vi "LSMcontroller_v62_updatedpointscan.vi"() -> ()   [LabVIEW 2015] (continued)
                                n1697 = call "calib.vi"() -> ()  [unwired: 1 in]
                                }
                                frame #2 {
                                n1698 = call "setup.vi"() -> ()  [unwired: 1 in]
                                }
                                }
                                }
                                }
                              }
                              frame Enabled {
                              }
                            }
                            n1699 = local write "64bit disabled"(TRUE ("64bit disabled")) -> ()
                          }
                          frame #2 {
                            n1700 = local read "save\ndata"() -> (w4480:bool)
                            n1701 = case shown="True" w4480 {
                              tunnel: w4481 -> [_ w4485]
                              frame False {
                              }
                              frame True {
                                n1702 = local read "filename prefix"() -> (w4483:string)
                                n1703 = local read "data dir"() -> (w4484:path)
                                n1704 = call "preparebinaryfiles.vi"("filename prefix"=w4483, "data dir"=w4484, "timestamp"=w4485) -> ("full-filename"=w4482:string)  [unwired: 1 in]
                                n1705 = local write "full-filename"(w4482) -> ()
                              }
                            }
                            n1706 = call "preptempbuffers_tt.vi"() -> ()  [unwired: 12 in]
                          }
                          frame #3 {
                            n1707 = local read "wavdet"() -> (w4486:bool)
                            n1708 = case shown="False" w4486 {
                              frame False {
                                n1709 = disable-structure shown="Disabled" {
                                frame Disabled {
                                n1710 = call "2pparameters.vi"("command"="get") -> ("params out"=w4488:T10)  [unwired: 1 in]
                                n1711 = Unbundle By Name(w4488) -> ("autoshutter"=w4489:bool)
                                n1712 = case shown="True" w4489 {
                                frame False {
                                }
                                frame True {
                                n1713 = call "shuttercontrol.vi"("command"="open") -> ()  [unwired: 1 in, 1 out]
                                }
                                }
                                }
                                frame Enabled {
                                }
                                }
                              }
                              frame True {
                              }
                            }
                          }
                          frame #4 {
                            n1714 = flat-sequence {
                              frame #0 {
                                # "Disabled for conversion to 64 bit"
                                n1715 = disable-structure shown="Disabled" {
                                frame Disabled {
                                n1716 = local read "Measurement"() -> (w4492:T4)
                                n1717 = case shown="\"Lifetime (contour)\"" w4492 {
                                frame "X-Y-t movie", Default {
                                }
                                frame "Lifetime (contour)" {
                                n1718 = call "runLT_img.vi"() -> ()  [unwired: 1 in]
                                }
                                }
                                }
                                frame Enabled {
                                }
                                }
                                n1719 = local write "64bit disabled"(TRUE ("64bit disabled")) -> ()
                              }
                              frame #1 {
                                n1720 = call "runAI_img.vi"() -> ()  [unwired: 12 in]
                                n1721 = call "runCI.vi"() -> ()  [unwired: 12 in]
                                n1722 = call "runDO_img.vi"() -> ()  [unwired: 12 in]
                              }
                              frame #2 {
                                n1723 = call "runAO_img.vi"() -> ()  [unwired: 12 in]
                              }
                            }
                          }
                          frame #5 {
                            # "Disabled for conversion to 64 bit"
                            n1724 = disable-structure shown="Disabled" {
                              disable-tunnel: w4494 -> [w4495 _]
                              frame Disabled {
                                w4498 = u16 0 items=["Stream to disk", "Post process", "real time process"] ("Ring")
                                n1725 = local read "T3R Data processing"() -> (w4497:u16)
                                n1726 = Equal?(x=w4497, y=w4498) -> (x = y?=w4496:bool)
                                n1727 = local read "save\ndata"() -> (w4500:bool)
                                n1728 = local read "Measurement"() -> (w4501:T4)
                                n1729 = And(x=w4500, y=w4496) -> (x .and. y?=w4499:bool)
                                n1730 = case shown="\"Lifetime (contour)\"" w4501 {
                                tunnel: w4495 -> [_ w4505]
                                tunnel: w4499 -> [_ w4503]
                                frame "X-Y-t movie", Default {
                                }
                                frame "Lifetime (contour)" {
                                n1731 = case shown="True" w4503 {
                                selector: w4503 -> [w4506 w4511]
                                tunnel: w4505 -> [_ w4509]
                                tunnel: [path "" ("appended path") w4512] -> w4504
                                tunnel: [w4506 w4511] -> w4502
                                frame False {
                                }
                                frame True {
                                n1732 = local read "filename prefix"() -> (w4510:string)
                                n1733 = local read "data dir"() -> (w4513:path)
                                n1734 = call "generatedatafilename.vi"("timestamp"=w4509, "filename prefix in"=w4510) -> ("full-filename"=w4508:string)
                                n1735 = Concatenate Strings(w4508, ".lvpt3contour" ("string")) -> (w4515:string)
                                n1736 = Build Path(base path=w4513, name or relative path=w4515) -> (appended path=w4512:path)
                                }
                                }
                                n1737 = call "collectLT_res_v1.vi"("stream?"=w4502, "data file"=w4504) -> ()  [unwired: 2 out]
                                }
                                }
                              }
                              frame Enabled {
                              }
                            }
                            n1738 = while {
                              i -> [w4518]
                              stop <- w4516 stop-if-true
                              n1739 = local read "Stop"() -> (w4526:bool)
                              n1740 = local read "Exit"() -> (w4525:bool)
                              n1741 = Increment(x=w4518) -> (x+1=w4517:i32)
                              n1742 = local write "points recorded"(w4517) -> ()
                              n1743 = Or(x=w4526, y=w4525) -> (x .or. y?=w4524:bool)
                              n1744 = case shown="False" w4524 {
                                frame False {
                                n1745 = stacked-sequence {
                                frame #0 {
                                n1746 = call "collectAI_tt_V2.vi"() -> ()  [unwired: 4 in]
                                n1747 = call "collectCI_tt.vi"() -> ("size(s)"=w4533:i32)  [unwired: 3 in]
                                n1748 = local write "scol"(w4533) -> ()
                                }
                                frame #1 {
                                n1749 = local read "Live"() -> (w4534:bool)
                                n1750 = case shown="True" w4534 {
                                frame False {
                                }
                                frame True {
                                n1751 = local read "graph1list"() -> (w4541:u16)
                                n1752 = local read "graph2list"() -> (w4540:u16)
                                n1753 = To Unsigned Word Integer(number=w4541) -> (unsigned 16bit integer=w4539:u16)
                                n1754 = To Unsigned Word Integer(number=w4540) -> (unsigned 16bit integer=w4538:u16)
                                n1755 = call "dattotrace.vi"("graph2list"=w4538, "Current Average"=sgl 1.0, "graph1list"=w4539) -> ("trace2array out"=w4536:sgl[], "trace1array out"=w4547:sgl[])
                                n1756 = local read "bin"() -> (w4548:dbl)
                                n1757 = script code="data=reshape(datain,[bin length(datain)./bin]);\ndataout=mean(data,1);\ndata2=reshape(datain2,[bin length(datain2)./bin]);\ndataout2=mean(data2,1);"("bin"=w4548, "datain"=w4547, "datain2"=w4536) -> ("dataout"=w4546:dbl[], "dataout2"=w4535:dbl[])  [unwired: 1 in, 1 out]
                                n1758 = Array Size(array=w4535) -> (size(s)=w4549:i32)
                                n1759 = Divide(x=w4549, y=2) -> (x/y=w4551:dbl)
                                n1760 = Round To Nearest(number=w4551) -> (nearest integer value=w4553:dbl)
                                n1761 = Array Size(array=w4546) -> (size(s)=w4558:i32)
                                n1762 = Delete From Array(array=w4535, length=w4553, index=0) -> (deleted portion=w4544:dbl[], array with subset deleted=w4545:dbl[])
                                n1763 = Divide(x=w4558, y=2) -> (x/y=w4556:dbl)
                                n1764 = Round To Nearest(number=w4556) -> (nearest integer value=w4554:dbl)
                                n1765 = Delete From Array(array=w4546, length=w4554, index=0) -> (deleted portion=w4543:dbl[], array with subset deleted=w4542:dbl[])
                                n1766 = local write "graph2"(w4542) -> ()
                                n1767 = local write "graph1"(w4543) -> ()
                                n1768 = local write "graph3"(w4544) -> ()
                                n1769 = local write "graph4"(w4545) -> ()
                                }
                                }
                                }
                                frame #2 {
                                n1770 = local read "save\ndata"() -> (w4559:bool)
                                n1771 = case shown="True" w4559 {
                                frame False {
                                }
                                frame True {
                                n1772 = call "savebinaryfiles.vi"() -> ()  [unwired: 1 in]
                                }
                                }
                                }
                                }
                                }
                                frame True {
                                }
                              }
                              n1773 = local read "continuous"() -> (w4521:bool)
                              n1774 = case shown="False" w4521 {
                                tunnel: w4517 -> [w4531 _]
                                tunnel: [w4530 FALSE] -> w4519
                                frame False {
                                n1775 = call "2pparameters.vi"("command"="get") -> ("params out"=w4528:T10)  [unwired: 1 in]
                                n1776 = Unbundle By Name(w4528) -> ("tt_cycles"=w4527:i32)
                                n1777 = Greater Or Equal?(x=w4531, y=w4527) -> (x >= y?=w4530:bool)
                                }
                                frame True {
                                }
                              }
                              n1778 = local read "Stop"() -> (w4523:bool)
                              n1779 = local read "Exit"() -> (w4522:bool)
                              n1780 = Or(x=w4523, y=w4522) -> (x .or. y?=w4520:bool)
                              n1781 = Or(x=w4520, y=w4519) -> (x .or. y?=w4516:bool)
                            }
                            n1782 = local write "64bit disabled"(TRUE ("64bit disabled")) -> ()
                          }
                          frame #6 {
                            # "Disabled for conversion to 64 bit"
                            n1783 = local read "Measurement"() -> (w4562:T4)
                            n1784 = disable-structure shown="Disabled" {
                              disable-tunnel: w4562 -> [w4564 _]
                              disable-tunnel: w4561 -> [w4563 _]
                              frame Disabled {
                                n1785 = case shown="\"Lifetime (contour)\"" w4564 {
                                tunnel: w4563 -> [_ w4565]
                                frame "X-Y-t movie", Default {
                                }
                                frame "Lifetime (contour)" {
                                n1786 = stacked-sequence {
                                tunnel: w4565 -> [_ w4566]
                                frame #0 {
                                n1787 = flat-sequence {
                                frame #0 {
                                n1788 = call "stoperaseLT_img.vi"() -> ()  [unwired: 1 in]
                                }
                                }
                                }
                                frame #1 {
                                w4569 = u16 0 items=["Stream to disk", "Post process", "real time process"] ("Ring")
                                n1789 = local read "T3R Data processing"() -> (w4568:u16)
                                n1790 = local read "save\ndata"() -> (w4571:bool)
                                n1791 = Equal?(x=w4568, y=w4569) -> (x = y?=w4567:bool)
                                n1792 = Not(x=w4567) -> (.not. x?=w4572:bool)
                                n1793 = And(x=w4571, y=w4572) -> (x .and. y?=w4570:bool)
                                n1794 = case shown="True" w4570 {
                                tunnel: w4566 -> [_ w4573]
                                frame False {
                                }
                                frame True {
                                n1795 = local read "filename prefix"() -> (w4574:string)
                                n1796 = local read "data dir"() -> (w4590:path)
                                n1797 = call "2pparameters.vi"("command"="get") -> ("params out"=w4585:T10)  [unwired: 1 in]
                                n1798 = call "generatedatafilename.vi"("timestamp"=w4573, "filename prefix in"=w4574) -> ("full-filename"=w4575:string)
                                n1799 = Unbundle By Name(w4585) -> ("srate"=w4583:sgl, "Pel"=w4582:sgl, "measpoints"=w4580:i32)
                                n1800 = Concatenate Strings(w4575, ".lvpt3contour" ("string")) -> (w4588:string)
                                n1801 = Build Path(base path=w4590, name or relative path=w4588) -> (appended path=w4587:path)
                                n1802 = To Unsigned Long Integer(number=w4583) -> (unsigned 32bit integer=w4584:u32)
                                n1803 = To Unsigned Long Integer(number=w4582) -> (unsigned 32bit integer=w4581:u32)
                                n1804 = To Unsigned Long Integer(number=w4580) -> (unsigned 32bit integer=w4579:u32)
                                n1805 = call "PH-temp-raw.vi"("command"="get") -> ("array out"=w4578:u32[])  [unwired: 1 in]
                                n1806 = Build Array (concatenate)(w4584, w4581, w4579, w4578) -> (w4577:u32[])
                                n1807 = Open/Create/Replace File(file path (use dialog)=w4587, operation (0:open)=T8."replace or create") -> (refnum out=w4594:refnum<file>, error out=w4593:errorcluster)  [unwired: 4 in, 1 out]
                                n1808 = Write to Binary File(file (use dialog)=w4594, data=w4577, error in=w4593, 5:FALSE ("prepend array or string size? (T)")) -> (refnum out=w4591:refnum<file>, error out=w4592:errorcluster)  [unwired: 2 in, 1 out]
                                n1809 = Close File(refnum=w4591, error in=w4592) -> ()  [unwired: 2 out]
                                }
                                }
                                }
                                }
                                }
                                }
                              }
                              frame Enabled {
                              }
                            }
                            n1810 = local write "64bit disabled"(TRUE ("64bit disabled")) -> ()
                          }
                          frame #7 {
                            n1811 = call "reset AO_DO_v3.vi"() -> ()  [unwired: 12 in]
                          }
                          frame #8 {
                            n1812 = stacked-sequence {
                              tunnel: w4610 -> [w4613 _ _ _ _ _]
                              tunnel: w4607 -> [w4612 _ _ _ _ _]
                              tunnel: w4608 -> [w4611 _ _ _ _ _]
                              tunnel: w4609 -> [_ w4662 _ _ _ _]
                              tunnel: w4605 -> [_ w4661 w4716 w4813 _ _]
                              tunnel: w4606 -> [_ w4660 w4715 w4812 _ _]
                              tunnel: w4604 -> [_ _ _ w4811 _ _]
                              tunnel: w4603 -> [_ _ _ w4810 _ _]
                              tunnel: w4602 -> [_ _ w4713 _ _ _]
                              tunnel: w4601 -> [_ _ w4712 _ _ _]
                              tunnel: w4600 -> [_ _ w4710 _ _ _]
                              tunnel: w4599 -> [_ _ w4709 _ _ _]
                              tunnel: w4598 -> [_ _ _ w4808 _ _]
                              tunnel: w4597 -> [_ _ _ w4807 _ _]
                              frame #0 {
                                n1813 = case shown="False" w4613 {
                                tunnel: w4612 -> [_ w4635]
                                tunnel: w4611 -> [_ w4634]
                                frame True {
                                n1814 = stacked-sequence {
                                seq-local: [w4614 _ _] -> [_ w4626 w4631]
                                frame #0 {
                                n1815 = call "configuration.vi"("command"="get") -> ("config out"=w4620:T11)  [unwired: 2 in, 1 out]
                                n1816 = Unbundle By Name(w4620) -> ("Voltage to Xgalvo"=w4617:i32)
                                n1817 = call "2pparameters.vi"("command"="get") -> ("params out"=w4618:T10)  [unwired: 1 in]
                                n1818 = in-place {
                                in-place-border: w4617 -> [w4625]
                                in-place-border: [w4622] -> w4614
                                n1819 = in-place-cluster #31(w4618) -> ("aAO"=w4624:u32[])
                                n1820 = call "remove channel from active arrayv2.vi"("line array in"=w4624, "line to remove"=w4625) -> ("line array out"=w4623:u32[], "index"=w4622:i32)  [unwired: 1 out]
                                n1821 = in-place-cluster #31("aAO"=w4623) -> (w4615:T10)
                                }
                                n1822 = call "2pparameters.vi"("Params in"=w4615, "command"="set") -> ()  [unwired: 1 out]
                                }
                                frame #1 {
                                n1823 = call "waveformparamsv2.vi"("command"="rem AO", "index"=w4626) -> ()  [unwired: 3 in, 3 out]
                                }
                                frame #2 {
                                n1824 = call "waveformsAObuffer.vi"("command"="get") -> ("AO wf out"=w4632:waveform(dbl)[])  [unwired: 1 in]
                                n1825 = Delete From Array(array=w4632, length=1, index=w4631) -> (array with subset deleted=w4628:waveform(dbl)[])  [unwired: 1 out]
                                n1826 = call "waveformsAObuffer.vi"("AO wf in"=w4628, "command"="set") -> ()  [unwired: 1 out]
                                }
                                }
                                }
                                frame False {
                                n1827 = stacked-sequence {
                                seq-local: [w4636 _ _] -> [_ w4644 w4655]
                                tunnel: w4635 -> [_ w4643 _]
                                tunnel: w4634 -> [_ _ w4654]
                                frame #0 {
                                n1828 = call "configuration.vi"("command"="get") -> ("config out"=w4641:T11)  [unwired: 2 in, 1 out]
                                n1829 = Unbundle By Name(w4641) -> ("Voltage to Xgalvo"=w4637:i32)
                                n1830 = call "2pparameters.vi"("command"="get") -> ("params out"=w4640:T10)  [unwired: 1 in]
                                n1831 = Unbundle By Name(w4640) -> ("aAO"=w4638:u32[])
                                n1832 = Search 1D Array(1D array=w4638, element=w4637) -> (index of element=w4636:i32)  [unwired: 1 in]
                                }
                                frame #1 {
                                n1833 = call "waveformparamsv2.vi"("command"="get") -> ("Params out"=w4647:T14)  [unwired: 4 in, 2 out]
                                n1834 = in-place {
                                in-place-border: w4644 -> [w4651]
                                in-place-border: w4643 -> [w4650]
                                n1835 = in-place-cluster #32(w4647) -> ("AO parameters"=w4652:T15)
                                n1836 = in-place {
                                in-place-border: w4650 -> [w4653]
                                n1837 = in-place-array #33(w4652, w4651) -> ()  [unwired: 1 out]
                                n1838 = in-place-array #33(w4653) -> (w4649:T15)  [unwired: 1 out]
                                }
                                n1839 = in-place-cluster #32("AO parameters"=w4649) -> (w4645:T14)
                                }
                                n1840 = call "waveformparamsv2.vi"("command"="set", "Params in"=w4645) -> ()  [unwired: 3 in, 3 out]
                                }
                                frame #2 {
                                n1841 = call "waveformsAObuffer.vi"("command"="get") -> ("AO wf out"=w4658:waveform(dbl)[])  [unwired: 1 in]
                                n1842 = Replace Array Subset(array=w4658, new element=w4654, index=w4655) -> (w4656:waveform(dbl)[])
                                n1843 = call "waveformsAObuffer.vi"("AO wf in"=w4656, "command"="set") -> ()  [unwired: 1 out]
                                }
                                }
                                }
                                }
                              }
                              frame #1 {
                                n1844 = case shown="False" w4662 {
                                tunnel: w4661 -> [_ w4684]
                                tunnel: w4660 -> [_ w4683]
                                frame True {
                                n1845 = stacked-sequence {
                                seq-local: [w4663 _ _] -> [_ w4675 w4680]
                                frame #0 {
                                n1846 = call "configuration.vi"("command"="get") -> ("config out"=w4669:T11)  [unwired: 2 in, 1 out]
                                n1847 = Unbundle By Name(w4669) -> ("Voltage to Ygalvo"=w4666:i32)
                                n1848 = call "2pparameters.vi"("command"="get") -> ("params out"=w4667:T10)  [unwired: 1 in]
                                n1849 = in-place {
                                in-place-border: w4666 -> [w4674]
                                in-place-border: [w4671] -> w4663
                                n1850 = in-place-cluster #34(w4667) -> ("aAO"=w4673:u32[])
                                n1851 = call "remove channel from active arrayv2.vi"("line array in"=w4673, "line to remove"=w4674) -> ("line array out"=w4672:u32[], "index"=w4671:i32)  [unwired: 1 out]
                                n1852 = in-place-cluster #34("aAO"=w4672) -> (w4664:T10)
                                }
                                n1853 = call "2pparameters.vi"("Params in"=w4664, "command"="set") -> ()  [unwired: 1 out]
                                }
                                frame #1 {
                                n1854 = call "waveformparamsv2.vi"("command"="rem AO", "index"=w4675) -> ()  [unwired: 3 in, 3 out]
                                }
                                frame #2 {
                                n1855 = call "waveformsAObuffer.vi"("command"="get") -> ("AO wf out"=w4681:waveform(dbl)[])  [unwired: 1 in]
                                n1856 = Delete From Array(array=w4681, length=1, index=w4680) -> (array with subset deleted=w4677:waveform(dbl)[])  [unwired: 1 out]
                                n1857 = call "waveformsAObuffer.vi"("AO wf in"=w4677, "command"="set") -> ()  [unwired: 1 out]
                                }
                                }
                                }
                                frame False {
                                n1858 = stacked-sequence {
                                seq-local: [w4685 _ _] -> [_ w4693 w4704]
                                tunnel: w4684 -> [_ w4692 _]
                                tunnel: w4683 -> [_ _ w4703]
                                frame #0 {
                                n1859 = call "configuration.vi"("command"="get") -> ("config out"=w4690:T11)  [unwired: 2 in, 1 out]
                                n1860 = Unbundle By Name(w4690) -> ("Voltage to Ygalvo"=w4686:i32)
                                n1861 = call "2pparameters.vi"("command"="get") -> ("params out"=w4689:T10)  [unwired: 1 in]
                                n1862 = Unbundle By Name(w4689) -> ("aAO"=w4687:u32[])
                                n1863 = Search 1D Array(1D array=w4687, element=w4686) -> (index of element=w4685:i32)  [unwired: 1 in]
                                }
                                frame #1 {
                                n1864 = call "waveformparamsv2.vi"("command"="get") -> ("Params out"=w4696:T14)  [unwired: 4 in, 2 out]
                                n1865 = in-place {
                                in-place-border: w4693 -> [w4700]
                                in-place-border: w4692 -> [w4699]
                                n1866 = in-place-cluster #35(w4696) -> ("AO parameters"=w4701:T15)
                                n1867 = in-place {
                                in-place-border: w4699 -> [w4702]
                                n1868 = in-place-array #36(w4701, w4700) -> ()  [unwired: 1 out]
                                n1869 = in-place-array #36(w4702) -> (w4698:T15)  [unwired: 1 out]
                                }
                                n1870 = in-place-cluster #35("AO parameters"=w4698) -> (w4694:T14)
                                }
                                n1871 = call "waveformparamsv2.vi"("command"="set", "Params in"=w4694) -> ()  [unwired: 3 in, 3 out]
                                }
                                frame #2 {
                                n1872 = call "waveformsAObuffer.vi"("command"="get") -> ("AO wf out"=w4707:waveform(dbl)[])  [unwired: 1 in]
                                n1873 = Replace Array Subset(array=w4707, new element=w4703, index=w4704) -> (w4705:waveform(dbl)[])
                                n1874 = call "waveformsAObuffer.vi"("AO wf in"=w4705, "command"="set") -> ()  [unwired: 1 out]
                                }
                                }
                                }
                                }
                              }
                              frame #2 {
                                n1875 = Build Array(w4713, w4712) -> (w4714:bool[])
                                n1876 = Boolean Array To Number(Boolean array=w4714) -> (number=w4711:u32)
                                n1877 = case shown="2" w4711 {
                                tunnel: w4716 -> [_ _ w4759]
                                tunnel: w4715 -> [_ _ w4758]
                                tunnel: w4710 -> [_ w4738 w4757]
                                tunnel: w4709 -> [_ w4737 w4756]
                                frame 1, Default {
                                n1878 = stacked-sequence {
                                seq-local: [w4717 _ _] -> [_ w4729 w4734]
                                frame #0 {
                                n1879 = call "configuration.vi"("command"="get") -> ("config out"=w4723:T11)  [unwired: 2 in, 1 out]
                                n1880 = Unbundle By Name(w4723) -> ("2P shutter"=w4720:i32)
                                n1881 = call "2pparameters.vi"("command"="get") -> ("params out"=w4721:T10)  [unwired: 1 in]
                                n1882 = in-place {
                                in-place-border: w4720 -> [w4728]
                                in-place-border: [w4725] -> w4717
                                n1883 = in-place-cluster #37(w4721) -> ("aDO"=w4727:u32[])
                                n1884 = call "remove channel from active arrayv2.vi"("line array in"=w4727, "line to remove"=w4728) -> ("line array out"=w4726:u32[], "index"=w4725:i32)  [unwired: 1 out]
                                n1885 = in-place-cluster #37("aDO"=w4726) -> (w4718:T10)
                                }
                                n1886 = call "2pparameters.vi"("Params in"=w4718, "command"="set") -> ()  [unwired: 1 out]
                                }
                                frame #1 {
                                n1887 = call "waveformparamsv2.vi"("command"="rem DO", "index"=w4729) -> ()  [unwired: 3 in, 3 out]
                                }
                                frame #2 {
                                n1888 = call "waveformsDObuffer.vi"("command"="get") -> ("DO wf out"=w4735:digitalwaveform[])  [unwired: 1 in]
                                n1889 = Delete From Array(array=w4735, length=1, index=w4734) -> (array with subset deleted=w4731:digitalwaveform[])  [unwired: 1 out]
                                n1890 = call "waveformsDObuffer.vi"("DO wf in"=w4731, "command"="set") -> ()  [unwired: 1 out]
                                }
                                }
                                }
                                frame 2 {
                                n1891 = stacked-sequence {
                                tunnel: w4738 -> [_ w4749 _]
                                tunnel: w4737 -> [_ _ w4751]
                                frame #0 {
                                n1892 = call "configuration.vi"("command"="get") -> ("config out"=w4740:T11)  [unwired: 2 in, 1 out]
                                n1893 = call "2pparameters.vi"("command"="get") -> ("params out"=w4744:T10)  [unwired: 1 in]
                                n1894 = Unbundle By Name(w4740) -> ("2P shutter"=w4739:i32)
                                n1895 = in-place {
                                in-place-border: w4739 -> [w4748]
                                n1896 = in-place-cluster #38(w4744) -> ("aDO"=w4747:u32[])
                                n1897 = call "add channel to active arrayv2.vi"("line array in"=w4747, "line to add"=w4748) -> ("line array out"=w4746:u32[])  [unwired: 2 out]
                                n1898 = in-place-cluster #38("aDO"=w4746) -> (w4742:T10)
                                }
                                n1899 = call "2pparameters.vi"("Params in"=w4742, "command"="set") -> ()  [unwired: 1 out]
                                }
                                frame #1 {
                                n1900 = call "waveformparamsv2.vi"("command"="add DO", "add DO"=w4749) -> ()  [unwired: 3 in, 3 out]
                                }
                                frame #2 {
                                n1901 = call "waveformsDObuffer.vi"("command"="get") -> ("DO wf out"=w4754:digitalwaveform[])  [unwired: 1 in]
                                n1902 = Build Array (concatenate)(w4754, w4751) -> (w4753:digitalwaveform[])
                                n1903 = call "waveformsDObuffer.vi"("DO wf in"=w4753, "command"="set") -> ()  [unwired: 1 out]
                                }
                                }
                                }
                                frame 0 {
                                n1904 = stacked-sequence {
                                seq-local: [w4760 _ _] -> [_ w4768 w4790]
                                tunnel: w4759 -> [_ _ _]
                                tunnel: w4758 -> [_ _ _]
                                tunnel: w4757 -> [_ w4767 _]
                                tunnel: w4756 -> [_ _ w4789]
                                frame #0 {
                                n1905 = call "configuration.vi"("command"="get") -> ("config out"=w4765:T11)  [unwired: 2 in, 1 out]
                                n1906 = call "2pparameters.vi"("command"="get") -> ("params out"=w4764:T10)  [unwired: 1 in]
                                n1907 = Unbundle By Name(w4765) -> ("2P shutter"=w4761:i32)
                                n1908 = Unbundle By Name(w4764) -> ("aDO"=w4762:u32[])
                                n1909 = Search 1D Array(1D array=w4762, element=w4761) -> (index of element=w4760:i32)  [unwired: 1 in]
                                }
                                frame #1 {
                                n1910 = call "2pparameters.vi"("command"="get") -> ("params out"=w4771:T10)  [unwired: 1 in]
                                n1911 = Unbundle By Name(w4771) -> ("wavdet"=w4769:bool, "autoshutter"=w4770:bool)
                                n1912 = case shown="True" w4770 {
                                tunnel: w4768 -> [_ w4775]
                                tunnel: w4769 -> [_ w4774]
                                tunnel: w4767 -> [_ w4773]
                                frame False {
                                }
                                frame True {
                                n1913 = case shown="False" w4774 {
                                tunnel: w4775 -> [w4779 _]
                                tunnel: w4773 -> [w4776 _]
                                frame False {
                                n1914 = Index Array(array=w4776, index=0) -> (element=w4777:T18)
                                n1915 = call "waveformparamsv2.vi"("command"="get") -> ("Params out"=w4782:T14)  [unwired: 4 in, 2 out]
                                n1916 = in-place {
                                in-place-border: w4779 -> [w4786]
                                in-place-border: w4777 -> [w4784]
                                n1917 = in-place-cluster #39(w4782) -> ("DO parameters"=w4787:T17)
                                n1918 = in-place {
                                in-place-border: w4784 -> [w4788]
                                n1919 = in-place-array #40(w4787, w4786) -> ()  [unwired: 1 out]
                                n1920 = in-place-array #40(w4788) -> (w4785:T17)  [unwired: 1 out]
                                }
                                n1921 = in-place-cluster #39("DO parameters"=w4785) -> (w4780:T14)
                                }
                                n1922 = call "waveformparamsv2.vi"("command"="set", "Params in"=w4780) -> ()  [unwired: 3 in, 3 out]
                                }
                                frame True {
                                }
                                }
                                }
                                }
                                }
                                frame #2 {
                                n1923 = call "2pparameters.vi"("command"="get") -> ("params out"=w4793:T10)  [unwired: 1 in]
                                n1924 = Unbundle By Name(w4793) -> ("wavdet"=w4791:bool, "autoshutter"=w4792:bool)
                                n1925 = case shown="True" w4792 {
                                tunnel: w4790 -> [_ w4797]
                                tunnel: w4791 -> [_ w4796]
                                tunnel: w4789 -> [_ w4795]
                                frame False {
                                }
                                frame True {
                                n1926 = case shown="False" w4796 {
                                tunnel: w4797 -> [w4801 _]
                                tunnel: w4795 -> [w4799 _]
                                frame False {
                                n1927 = Index Array(array=w4799, index=0) -> (element=w4798:digitalwaveform)
                                n1928 = call "waveformsDObuffer.vi"("command"="get") -> ("DO wf out"=w4803:digitalwaveform[])  [unwired: 1 in]
                                n1929 = Replace Array Subset(array=w4803, new element=w4798, index=w4801) -> (w4805:digitalwaveform[])
                                n1930 = call "waveformsDObuffer.vi"("DO wf in"=w4805, "command"="set") -> ()  [unwired: 1 out]
                                }
                                frame True {
                                }
                                }
                                }
                                }
                                }
                                }
                                }
                                }
                              }
                              frame #3 {
                                n1931 = Build Array(w4808, w4807) -> (w4809:bool[])
                                n1932 = Boolean Array To Number(Boolean array=w4809) -> (number=w4806:u32)
                                n1933 = case shown="2" w4806 {
                                tunnel: w4813 -> [_ _ w4856]
                                tunnel: w4812 -> [_ _ w4855]
                                tunnel: w4811 -> [_ w4835 w4853]
                                tunnel: w4810 -> [_ w4834 w4854]
                                frame 1, Default {
                                n1934 = stacked-sequence {
                                seq-local: [w4814 _ _] -> [_ w4826 w4831]
                                frame #0 {
                                n1935 = call "configuration.vi"("command"="get") -> ("config out"=w4820:T11)  [unwired: 2 in, 1 out]
                                n1936 = Unbundle By Name(w4820) -> ("LT timestamp"=w4817:u32)
                                n1937 = call "2pparameters.vi"("command"="get") -> ("params out"=w4818:T10)  [unwired: 1 in]
                                n1938 = in-place {
                                in-place-border: w4817 -> [w4825]
                                in-place-border: [w4822] -> w4814
                                n1939 = in-place-cluster #41(w4818) -> ("aDO"=w4824:u32[])
                                n1940 = call "remove channel from active arrayv2.vi"("line array in"=w4824, "line to remove"=w4825) -> ("line array out"=w4823:u32[], "index"=w4822:i32)  [unwired: 1 out]
                                n1941 = in-place-cluster #41("aDO"=w4823) -> (w4815:T10)
                                }
                                n1942 = call "2pparameters.vi"("Params in"=w4815, "command"="set") -> ()  [unwired: 1 out]
                                }
                                frame #1 {
                                n1943 = call "waveformparamsv2.vi"("command"="rem DO", "index"=w4826) -> ()  [unwired: 3 in, 3 out]
                                }
                                frame #2 {
                                n1944 = call "waveformsDObuffer.vi"("command"="get") -> ("DO wf out"=w4832:digitalwaveform[])  [unwired: 1 in]
                                n1945 = Delete From Array(array=w4832, length=1, index=w4831) -> (array with subset deleted=w4828:digitalwaveform[])  [unwired: 1 out]
                                n1946 = call "waveformsDObuffer.vi"("DO wf in"=w4828, "command"="set") -> ()  [unwired: 1 out]
                                }
                                }
                                }
                                frame 2 {
                                n1947 = stacked-sequence {
                                tunnel: w4835 -> [_ _ w4848]
                                tunnel: w4834 -> [_ w4846 _]
                                frame #0 {
                                n1948 = call "configuration.vi"("command"="get") -> ("config out"=w4837:T11)  [unwired: 2 in, 1 out]
                                n1949 = Unbundle By Name(w4837) -> ("LT timestamp"=w4836:u32)
                                n1950 = call "2pparameters.vi"("command"="get") -> ("params out"=w4841:T10)  [unwired: 1 in]
                                n1951 = in-place {
                                in-place-border: w4836 -> [w4845]
                                n1952 = in-place-cluster #42(w4841) -> ("aDO"=w4844:u32[])
                                n1953 = call "add channel to active arrayv2.vi"("line array in"=w4844, "line to add"=w4845) -> ("line array out"=w4843:u32[])  [unwired: 2 out]
                                n1954 = in-place-cluster #42("aDO"=w4843) -> (w4839:T10)
                                }
                                n1955 = call "2pparameters.vi"("Params in"=w4839, "command"="set") -> ()  [unwired: 1 out]
                                }
                                frame #1 {
                                n1956 = call "waveformparamsv2.vi"("command"="add DO", "add DO"=w4846) -> ()  [unwired: 3 in, 3 out]
                                }
                                frame #2 {
                                n1957 = call "waveformsDObuffer.vi"("command"="get") -> ("DO wf out"=w4851:digitalwaveform[])  [unwired: 1 in]
                                n1958 = Build Array (concatenate)(w4851, w4848) -> (w4850:digitalwaveform[])
                                n1959 = call "waveformsDObuffer.vi"("DO wf in"=w4850, "command"="set") -> ()  [unwired: 1 out]
                                }
                                }
                                }
                                frame 0 {
                                n1960 = stacked-sequence {
                                seq-local: [w4857 _ _] -> [_ w4867 w4884]
                                tunnel: w4856 -> [_ _ _]
                                tunnel: w4855 -> [_ _ _]
                                tunnel: w4854 -> [_ w4864 _]
                                tunnel: w4853 -> [_ _ w4883]
                                frame #0 {
                                n1961 = call "configuration.vi"("command"="get") -> ("config out"=w4862:T11)  [unwired: 2 in, 1 out]
                                n1962 = Unbundle By Name(w4862) -> ("LT timestamp"=w4858:u32)
                                n1963 = call "2pparameters.vi"("command"="get") -> ("params out"=w4861:T10)  [unwired: 1 in]
                                n1964 = Unbundle By Name(w4861) -> ("aDO"=w4859:u32[])
                                n1965 = Search 1D Array(1D array=w4859, element=w4858) -> (index of element=w4857:i32)  [unwired: 1 in]
                                }
                                frame #1 {
                                n1966 = local read "Measurement"() -> (w4866:T4)
                                n1967 = To Unsigned Long Integer(number=w4866) -> (unsigned 32bit integer=w4865:u32)
                                n1968 = case shown="5..7" w4865 {
                                tunnel: w4867 -> [_ w4871]
                                tunnel: w4864 -> [_ w4868]
                                frame 0..4, Default {
                                }
                                frame 5..7 {
                                n1969 = Index Array(array=w4868, index=0) -> (element=w4869:T18)
                                n1970 = call "waveformparamsv2.vi"("command"="get") -> ("Params out"=w4874:T14)  [unwired: 4 in, 2 out]
                                n1971 = in-place {
                                in-place-border: w4871 -> [w4878]
                                in-place-border: w4869 -> [w4876]
                                n1972 = in-place-cluster #43(w4874) -> ("DO parameters"=w4879:T17)
                                n1973 = in-place {
                                in-place-border: w4876 -> [w4880]
                                n1974 = in-place-array #44(w4879, w4878) -> ()  [unwired: 1 out]
                                n1975 = in-place-array #44(w4880) -> (w4877:T17)  [unwired: 1 out]
                                }
                                n1976 = in-place-cluster #43("DO parameters"=w4877) -> (w4872:T14)
                                }
                                n1977 = call "waveformparamsv2.vi"("command"="set", "Params in"=w4872) -> ()  [unwired: 3 in, 3 out]
                                }
                                }
                                }
                                frame #2 {
                                n1978 = local read "Measurement"() -> (w4882:T4)
                                n1979 = To Unsigned Long Integer(number=w4882) -> (unsigned 32bit integer=w4881:u32)
                                n1980 = case shown="5..7" w4881 {
                                tunnel: w4884 -> [_ w4888]
                                tunnel: w4883 -> [_ w4886]
                                frame 0..4, Default {
                                }
                                frame 5..7 {
                                n1981 = Index Array(array=w4886, index=0) -> (element=w4885:digitalwaveform)
                                n1982 = call "waveformsDObuffer.vi"("command"="get") -> ("DO wf out"=w4890:digitalwaveform[])  [unwired: 1 in]
                                n1983 = Replace Array Subset(array=w4890, new element=w4885, index=w4888) -> (w4892:digitalwaveform[])
                                n1984 = call "waveformsDObuffer.vi"("DO wf in"=w4892, "command"="set") -> ()  [unwired: 1 out]
                                }
                                }
                                }
                                }
                                }
                                }
                              }
                              frame #4 {
                                n1985 = call "Used AO lines.vi"() -> ("used AO names"=w4895:string[], "used AO lines"=w4893:tag[])  [unwired: 2 in]
                                n1986 = control-ref of="Analog Lines Plot"() -> (w4894:refnum<vi>)
                                n1987 = control-ref of="Digital Lines Plot"() -> (w4896:refnum<vi>)
                                n1988 = call "Used DO lines.vi"() -> ("used DO names"=w4897:string[], "used DO lines"=w4898:tag[])  [unwired: 2 in]
                                n1989 = local write "Analog Used Lines"(w4893) -> ()
                                n1990 = local write "Analog Used Names"(w4895) -> ()
                                n1991 = local write "Digital Used Lines"(w4898) -> ()
                                n1992 = local write "Digital Used Names"(w4897) -> ()
                                n1993 = call "prepDOWaveplot.vi"("DigitalGraph in"=w4896, "used DO names"=w4897) -> ()  [unwired: 1 in]
                                n1994 = call "prepAOWaveplot.vi"("WaveformGraph in"=w4894, "Analog Used Names"=w4895) -> ()  [unwired: 1 in]
                              }
                              frame #5 {
                                n1995 = local read "Meastab"() -> (w4913:enum32{"X-Y Image", "Linescan", "Timetrace"})
                                n1996 = property on="refwf" class="Ring (strict)"() -> ("RingText.Text"=w4910:string)  [unwired: 2 in, 2 out]
                                n1997 = case shown="\"Timetrace\"" w4913 {
                                tunnel: [w4915 w4916] -> w4914
                                frame "X-Y Image", Default {
                                n1998 = local read "Sampling rate"() -> (w4915:dbl)
                                }
                                frame "Timetrace" {
                                n1999 = local read "srateAODOtt"() -> (w4916:dbl)
                                }
                                }
                                n2000 = call "waveformsAObuffer.vi"("command"="get") -> ("AO wf out"=w4901:waveform(dbl)[])  [unwired: 1 in]
                                n2001 = local read "wavdet"() -> (w4911:bool)
                                n2002 = call "waveformsDObuffer.vi"("command"="get") -> ("DO wf out"=w4905:digitalwaveform[])  [unwired: 1 in]
                                n2003 = call "correctwaveformsizetemp.vi"("new sampling frequency (Hz)"=w4914, "start"=FALSE, "reference waveforms to"=w4910, "Analog waveforms in"=w4901, "stop"=TRUE, "Digital waveforms in"=w4905) -> ("analog wf out"=w4907:waveform(dbl)[], "Digital wf out"=w4909:digitalwaveform[], "measpoints"=w4912:i32)
                                n2004 = local write "Analog Lines Plot"(w4907) -> ()
                                n2005 = call "GetNumCamFramesv2.vi"("Digital Waveform Graph"=w4909) -> ("Numeric"=w4908:i32)  [unwired: 10 in]
                                n2006 = local write "Digital Lines Plot"(w4909) -> ()
                                n2007 = call "waveformsDObuffer.vi"("DO wf in"=w4909, "command"="set") -> ()  [unwired: 1 out]
                                n2008 = call "waveformsAObuffer.vi"("AO wf in"=w4907, "command"="set") -> ()  [unwired: 1 out]
                                n2009 = local write "Total Camera Frames"(w4908) -> ()
                                n2010 = case shown="True" w4911 {
                                tunnel: w4912 -> [_ w4917]
                                frame False {
                                }
                                frame True {
                                n2011 = local write "# of frames"(w4917) -> ()
                                }
                                }
                              }
                            }
                            n2012 = call "stoperaseCI.vi"() -> ()  [unwired: 12 in]
                            n2013 = call "stoperaseDO_img.vi"() -> ()  [unwired: 12 in]
                            n2014 = call "stoperaseAO_img.vi"() -> ()  [unwired: 12 in]
                            n2015 = call "stoperaseAI_img.vi"() -> ()  [unwired: 12 in]
                          }
                          frame #9 {
                            w4927 = FALSE ("Value (Signaling)")
                            n2016 = local read "save\ndata"() -> (w4922:bool)
                            n2017 = case shown="True" w4922 {
                              tunnel: w4921 -> [_ w4934]
                              frame False {
                              }
                              frame True {
                                n2018 = call "closebinaryfiles.vi"() -> ()  [unwired: 12 in]
                                n2019 = local read "filename prefix"() -> (w4936:string)
                                n2020 = local read "data dir"() -> (w4935:path)
                                n2021 = call "saveparams.vi"("timestamp"=w4934, "filename prefix in"=w4936, "data dir in"=w4935) -> ()  [unwired: 1 in]
                              }
                            }
                            n2022 = call "2pparameters.vi"("command"="get") -> ("params out"=w4918:T10)  [unwired: 1 in]
                            n2023 = Unbundle By Name(w4918) -> ("auto OD"=w4919:bool)
                            n2024 = case shown="True" w4919 {
                              frame False {
                              }
                              frame True {
                                n2025 = call "configuration.vi"("command"="get") -> ("config out"=w4930:T11)  [unwired: 2 in, 1 out]
                                n2026 = call "2pparameters.vi"("command"="get") -> ("params out"=w4933:T10)  [unwired: 1 in]
                                n2027 = Unbundle By Name(w4930) -> ("contour OD"=w4928:u16)
                                n2028 = Unbundle By Name(w4933) -> ("ODfilt"=w4929:u16)
                                n2029 = call "filterwheelcontrol_nothorlabslib.vi"("Current OD filt"=w4928, "New ODfilt"=w4929) -> ()  [unwired: 1 in]
                              }
                            }
                            n2030 = property on="Start" class="Bool (strict)"("Val(Sgnl)"=w4927) -> ()  [unwired: 2 in, 2 out]
                            n2031 = property on="Start" class="Bool (strict)"("Visible"=TRUE, "DisabledEnum"=T7."Enabled" ("Disabled")) -> ()  [unwired: 2 in, 2 out]
                            n2032 = property on="Stop" class="Bool (strict)"("Val(Sgnl)"=w4927) -> ()  [unwired: 2 in, 2 out]
                            n2033 = property on="Stop" class="Bool (strict)"("Visible"=FALSE, "DisabledEnum"=T7."Disabled" ("Disabled")) -> ()  [unwired: 2 in, 2 out]
                          }
                          frame #10 {
                            w4939 = T21 2 items=["no dialog", "OK message", "continue or stop message", "OK message + warnings", "continue/stop + warnings"] ("type of dialog (OK msg:1)")
                            n2034 = call "displayerrors.vi"() -> ("error IO"=w4940:errorcluster)
                            n2035 = call <vilib>:"General Error Handler.vi"("type of dialog (OK msg:1)"=w4939, "error in (no error)"=w4940) -> ("error out"=w4938:errorcluster)  [unwired: 9 in, 4 out]
                            n2036 = call <vilib>:"Clear Errors.vi"("error in (no error)"=w4938) -> ("error out"=w4937:errorcluster)  [unwired: 5 in, 1 out]
                            n2037 = call "seterrors.vi"("error IO"=w4937) -> ()
                          }
                        }
                      }
                    }
                  }
                  frame "Lifetime (point)" {
                    # "Disabled for conversion to 64 bit"
                    n2038 = disable-structure shown="Disabled" {
                      frame Disabled {
                        n2039 = stacked-sequence {
                          frame #0 {
                            w4951 = 12.5 ("x")
                            # "get from syncrate"
                            n2040 = local read "Bin size"() -> (w4945:T6)
                            n2041 = local read "Vx-ref"() -> (w4957:dbl)
                            n2042 = local read "Vy-ref"() -> (w4958:dbl)
                            n2043 = call "2pparameters.vi"("command"="get") -> ("params out"=w4943:T10)  [unwired: 1 in]
                            n2044 = Scale By Power Of 2(n=w4945, x=1.0 ("Y Scale.Range:Minimum")) -> (x*2^n=w4954:dbl)
                            n2045 = call "setposition.vi"("Vy"=w4958, "Vx"=w4957) -> ()  [unwired: 1 in]
                            n2046 = Unbundle By Name(w4943) -> ("autoshutter"=w4944:bool)
                            n2047 = Multiply(x=3000.0 ("Y Scale.Range:Minimum"), y=w4954) -> (x*y=w4952:dbl)
                            n2048 = Compound Arithmetic op=MULTIPLY(w4951, invert 3200.0 ("X Scale.Offset and Multiplier:Multiplier"), w4954) -> (w4953:dbl)
                            n2049 = case shown="True" w4944 {
                              frame False {
                              }
                              frame True {
                                n2050 = call "shuttercontrol.vi"("command"="open") -> ()  [unwired: 1 in, 1 out]
                              }
                            }
                            n2051 = call "lifetimeparameters.vi"("command"="get") -> ("Params out"=w4949:T19)  [unwired: 1 in]
                            n2052 = property on="Histogram" class="WFGraph (strict)"("XScale.Maximum"=w4951, "XScale.Minimum"=0.0 ("X Scale.Range:Minimum"), "YScale.Maximum"=w4952, "YScale.Minimum"=0.1 ("Y Scale.Range:Minimum"), "XScale.Multiplier"=w4953) -> ()  [unwired: 2 in, 2 out]
                            n2053 = Bundle By Name(cluster=w4949, "Bin size"=w4945) -> (w4950:T19)
                            n2054 = call "lifetimeparameters.vi"("Params in"=w4950, "command"="set") -> ()  [unwired: 1 out]
                            n2055 = property on="Histogram 2" class="WFGraph (strict)"("YScale.Maximum"=w4952, "XScale.Multiplier"=w4953, "XScale.Maximum"=w4951) -> ()  [unwired: 2 in, 2 out]
                            n2056 = call "2pparameters.vi"("command"="get") -> ("params out"=w4965:T10)  [unwired: 1 in]
                            n2057 = Bundle By Name(cluster=w4965, "type"="Lifetime (point)") -> (w4963:T10)
                            n2058 = property on="Stop" class="Bool (strict)"("Visible"=TRUE, "DisabledEnum"=T7."Enabled" ("Disabled")) -> ()  [unwired: 2 in, 2 out]
                            n2059 = property on="Start" class="Bool (strict)"("Visible"=FALSE, "DisabledEnum"=T7."Disabled and Grayed Out" ("Disabled")) -> ()  [unwired: 2 in, 2 out]
                            n2060 = call "2pparameters.vi"("Params in"=w4963, "command"="set") -> ()  [unwired: 1 out]
                          }
                          frame #1 {
                            n2061 = call "setup.vi"() -> ()  [unwired: 1 in]
                          }
                          frame #2 {
                            # "main loop"
                            n2062 = call "lifetimeparameters.vi"("command"="get") -> ("Params out"=w4975:T19)  [unwired: 1 in]
                            n2063 = Unbundle By Name(w4975) -> ("devidx"=w4973:i32)
                            n2064 = for {
                              N: 10000 -> [_]
                              tunnel: [w4976] -> w4971 mode=indexing
                              i -> [w4976]
                            }
                            n2065 = while {
                              tunnel: w4973 -> [w4980]
                              tunnel: w4971 -> [w4977]
                              i -> [w4978]
                              stop <- w4982 stop-if-true
                              n2066 = Increment(x=w4978) -> (x+1=w4979:i32)
                              n2067 = dll-call lib="phlib.dll" fn="_PH_GetCountRate@8" label="PH_GetCountRate"("devidx"=w4980, "channel"=0) -> (w4981:i32)  [unwired: 5 in, 2 out]
                              "SyncRate" <- w4981
                              n2068 = stacked-sequence {
                                seq-local: [_ _ w4989 _ _] -> [_ _ _ w5002 _]
                                seq-local: [_ _ w4988 _ _] -> [_ _ _ w5001 _]
                                seq-local: [_ w4986 _ _ _] -> [_ _ w4990 _ _]
                                tunnel: w4981 -> [_ _ _ w5009 _]
                                tunnel: w4977 -> [_ _ _ w4999 _]
                                frame #0 {
                                n2069 = call "start_binned.vi"() -> ()  [unwired: 1 in]
                                }
                                frame #1 {
                                n2070 = call "get-histogram.vi"() -> ("IntegralCount"=→"Integral count":u32, "Histogram"=w4986:u32[])
                                "Histogram" <- w4986
                                }
                                frame #2 {
                                n2071 = Search 1D Array(1D array=w4990, element=u32 0) -> (index of element=w4988:i32)  [unwired: 1 in]
                                n2072 = Multiply(x=w4988, y=0.99) -> (x*y=w4994:dbl)
                                n2073 = Array Subset(array=w4990, index=0, length=w4994) -> (w4997:u32[])
                                n2074 = Array Max & Min(array=w4997) -> (max index (indices)=w4991:i32)  [unwired: 3 out]
                                n2075 = Split 1D Array(array=w4997, index=w4991) -> (second subarray=w4993:u32[])  [unwired: 1 out]
                                n2076 = Array Max & Min(array=w4993) -> (min index (indices)=w4992:i32)  [unwired: 3 out]
                                n2077 = Split 1D Array(array=w4993, index=w4992) -> (first subarray=w4989:u32[])  [unwired: 1 out]
                                "Histogram 2" <- w4989
                                }
                                frame #3 {
                                n2078 = Array Size(array=w5002) -> (size(s)=w5004:i32)
                                n2079 = Array Subset(array=w4999, index=0, length=w5004) -> (w5003:i32[])
                                n2080 = Compound Arithmetic op=MULTIPLY(1000000000.0 ("value"), invert w5009, invert w5001, w5003) -> (w5000:dbl[])
                                n2081 = call <vilib>:"Exponential Fit.vi"("Y"=w5002, "X"=w5000) -> ("damping"=w5006:dbl)  [unwired: 8 in, 5 out]
                                n2082 = Divide(x=-1.0 ("y"), y=w5006) -> (x/y=→"Lifetime (ns)":dbl)
                                }
                                frame #4 {
                                n2083 = local read "downright"() -> (w5016:bool)
                                n2084 = local read "downleft"() -> (w5018:bool)
                                n2085 = local read "upright"() -> (w5014:bool)
                                n2086 = local read "upleft"() -> (w5012:bool)
                                n2087 = local read "down"() -> (w5017:bool)
                                n2088 = local read "right"() -> (w5015:bool)
                                n2089 = local read "left"() -> (w5019:bool)
                                n2090 = local read "up"() -> (w5013:bool)
                                n2091 = Compound Arithmetic op=OR(w5012, w5013, w5014, w5015, w5016, w5017, w5018, w5019) -> (w5011:bool)
                                n2092 = case shown="True" w5011 {
                                frame False {
                                }
                                frame True {
                                n2093 = stacked-sequence {
                                frame #0 {
                                n2094 = local read "downright"() -> (w5021:bool)
                                n2095 = local read "downleft"() -> (w5023:bool)
                                n2096 = local read "BigSmall"() -> (w5020:bool)
                                n2097 = local read "upright"() -> (w5025:bool)
                                n2098 = local read "upleft"() -> (w5028:bool)
                                n2099 = local read "down"() -> (w5024:bool)
                                n2100 = local read "right"() -> (w5026:bool)
                                n2101 = local read "left"() -> (w5022:bool)
                                n2102 = local read "up"() -> (w5027:bool)
                                n2103 = call "movestageparams.vi"("command"="get") -> ("Params out"=w5031:T20)  [unwired: 1 in]
                                n2104 = Bundle By Name(cluster=w5031, "upleft"=w5028, "up"=w5027, "upright"=w5025, "right"=w5026, "downright"=w5021, "down"=w5024, "downleft"=w5023, "left"=w5022, "Bigsmall"=w5020) -> (w5032:T20)
                                n2105 = call "movestageparams.vi"("Params in"=w5032, "command"="set") -> ()  [unwired: 1 out]
                                }
                                frame #1 {
                                n2106 = call "movestage.vi"() -> ()  [unwired: 12 in]
                                }
                                frame #2 {
                                w5033 = FALSE ("OK Button")
                                w5034 = FALSE ("OK Button")
